vi "Gyro Color Assisted PID C1C2.vi"(4 "Colour 1 threshold":sgl=14.0, 6 "Ini. Degrees":sgl, 7 "Motor":cluster{"Port":T2, "Port":T2}={"Port"=1, "Port"=2} {"Port" items=["Port A", "Port B", "Port C", "Port D"]; "Port" items=["Port A", "Port B", "Port C", "Port D"]}, 9 "De-acc":i32=40, 10 "Acc":i32=80, 11 "EV3 in":T1) -> (3 "EV3 out":T1)   [LabVIEW 2016]
uses:
  <vilib>/NXT/Block Support/NXT_OutputPort.ctl
  <vilib>/NXT/Subs/LVHSConnector.ctl
  <vilib>/NXT/LegoClasses/BrickReference/BrickReference.lvclass
  <vilib>/NXT/Block Support/NXT_InputPort.ctl
  <vilib>/NXT/NXTIO Xnodes/NXTIONodeSubVIs/LEGOResetMotors.vi
  <vilib>/NXT/Dual Mode Library/Sensors/EV3_Gyro_Angle.vi
  <vilib>/NXT/Dual Mode Library/Motors/Rotation.vi
  <vilib>/NXT/Dual Mode Library/Sensors/EV3_Color_Reflect.vi
  <vilib>/NXT/NXTIO Xnodes/NXTIONodeSubVIs/NXTMotorSteeringOn.vi
  <vilib>/NXT/NXTIO Xnodes/NXTIOXNode/NXTIO.xnode
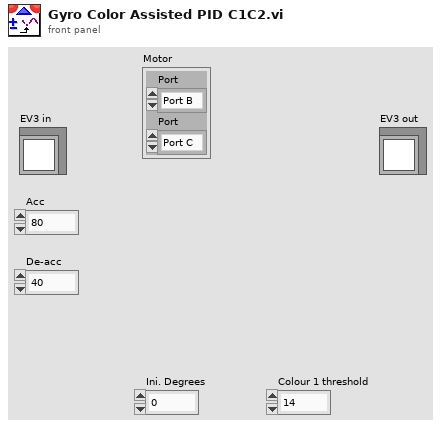
[diagram p1: front panel]
types:
  T1 = typedef "LVHSConnector.ctl" = refnum<class "BrickReference.lvclass">
  T2 = typedef "NXT_OutputPort.ctl" = u8
  T3 = typedef "NXT_InputPort.ctl" = u32
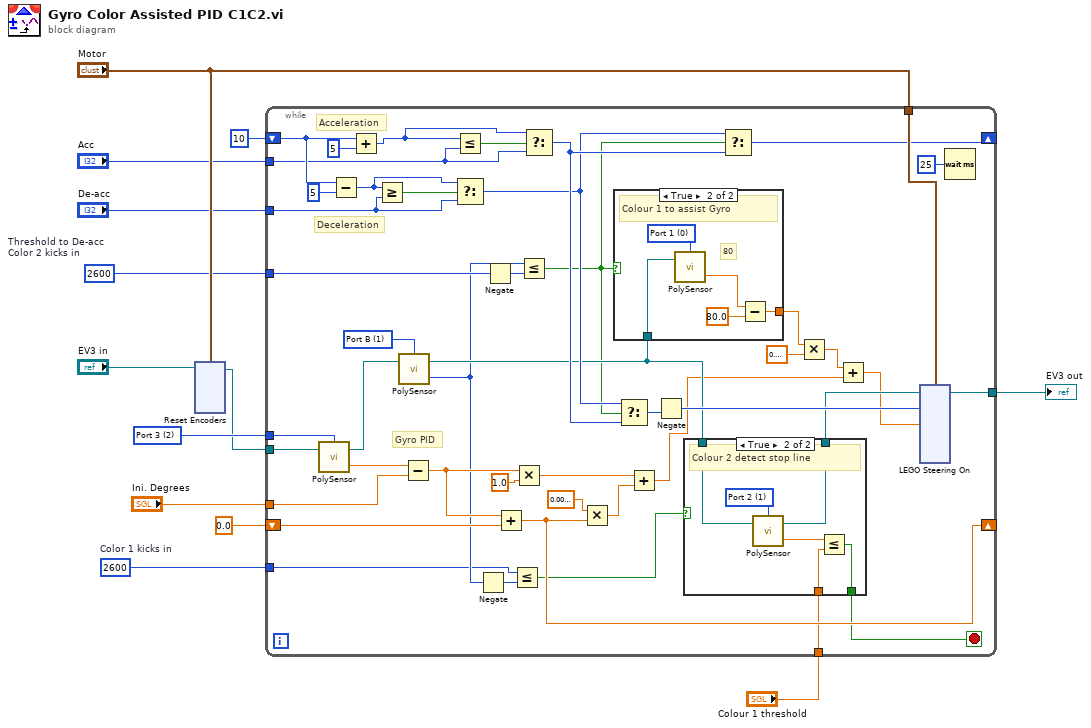
[diagram p0: block diagram]
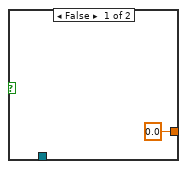
[diagram p2: hidden frame]
diagram:
  w1 = 2600  # Color 1 kicks in
  w3 = 2600  # Threshold to De-acc Color 2 kicks in
  w11 = T3 2 items=["Port 1", "Port 2", "Port 3", "Port 4"] ("Port (Gyro)")
  n1 = xnode "Reset Encoders"("Motors"="Motor", "NXT/EV3"="EV3 in") -> ("NXT/EV3"=w8:T1)
  n2 = while {
    tunnel: w8 -> [w50]
    tunnel: w11 -> [w44]
    shift-right: [w56] -> _
    shift-left: sgl 0.0 -> [w57]
    tunnel: "Ini. Degrees" -> [w52]
    tunnel: [w43] -> w2
    tunnel: "Motor" -> [w49]
    shift-right: [w29] -> _
    shift-left: 10 -> [w34]
    tunnel: "Colour 1 threshold" -> [w28]
    tunnel: "De-acc" -> [w27]
    tunnel: "Acc" -> [w26]
    tunnel: w3 -> [w19]
    tunnel: w1 -> [w14]
    stop <- w36 stop-if-true
    w47 = T2 1 items=["Port A", "Port B", "Port C", "Port D"] ("Port (Port A)")
    # "Acceleration"
    # "Gyro PID"
    # "Deceleration"
    n3 = call-poly <vilib>:"PolySensor.vi"("NXT/EV3"=w50, "Port (Port 1)"=w44) -> ("Degrees"=w59:sgl, "NXT/EV3"=w48:T1)  [unwired: 1 in]
    n4 = Subtract(x=w34, y=5) -> (x-y=w37:i32)
    n5 = Add(x=w34, y=5) -> (x+y=w32:i32)
    n6 = Greater Or Equal?(x=w37, y=w27) -> (x >= y?=w38:bool)
    n7 = call-poly <vilib>:"PolySensor.vi"("NXT/EV3"=w48, "Port (Port A)"=w47) -> ("Angle of Rotation"=w16:i32, "NXT/EV3"=w25:T1)  [unwired: 1 in]
    n8 = Subtract(x=w59, y=w52) -> (x-y=w51:sgl)
    n9 = Less Or Equal?(x=w32, y=w26) -> (x <= y?=w41:bool)
    n10 = Select(t=w37, s=w38, f=w27) -> (s? t:f=w30:i32)
    n11 = Negate(x=w16) -> (-x=w17:i32)
    n12 = Negate(x=w19) -> (-x=w45:i32)
    n13 = Add(x=w51, y=w57) -> (x+y=w56:sgl)
    n14 = Less Or Equal?(x=w14, y=w17) -> (x <= y?=w15:bool)
    n15 = Multiply(x=w51, y=sgl 1.0 ("K_p")) -> (x*y=w54:sgl)
    n16 = Less Or Equal?(x=w16, y=w45) -> (x <= y?=w18:bool)
    n17 = Select(t=w32, s=w41, f=w26) -> (s? t:f=w31:i32)
    n18 = Multiply(x=sgl 0.01 ("K_i"), y=w56) -> (x*y=w53:sgl)
    n19 = case shown="True" w18 {
      tunnel: w25 -> [_ w64]
      tunnel: [sgl 0.0 w63] -> w24
      frame False {
      }
      frame True {
        w65 = T3 0 items=["Port 1", "Port 2", "Port 3", "Port 4"] ("Port (Port 1)")
        # "80"
        # "Colour 1 to assist Gyro"
        n20 = call-poly <vilib>:"PolySensor.vi"("NXT/EV3"=w64, "Port (Port 1)"=w65) -> ("Scaled Value"=w61:sgl)  [unwired: 1 in, 1 out]
        n21 = Subtract(x=w61, y=sgl 80.0) -> (x-y=w63:sgl)
      }
    }
    n22 = Select(t=w30, s=w18, f=w31) -> (s? t:f=w40:i32)
    n23 = Add(x=w54, y=w53) -> (x+y=w21:sgl)
    n24 = Negate(x=w40) -> (-x=w46:i32)
    n25 = case shown="True" w15 {
      tunnel: [_ w70] -> w36
      tunnel: w25 -> [w66 w69]
      tunnel: [w66 w68] -> w35
      tunnel: w28 -> [_ w67]
      frame False {
      }
      frame True {
        w72 = T3 1 items=["Port 1", "Port 2", "Port 3", "Port 4"] ("Port (Port 1)")
        # "Colour 2 detect stop line"
        n26 = call-poly <vilib>:"PolySensor.vi"("NXT/EV3"=w69, "Port (Port 1)"=w72) -> ("Scaled Value"=w71:sgl, "NXT/EV3"=w68:T1)  [unwired: 1 in]
        n27 = Less Or Equal?(x=w71, y=w67) -> (x <= y?=w70:bool)
      }
    }
    n28 = Select(t=w30, s=w18, f=w31) -> (s? t:f=w29:i32)
    n29 = Multiply(x=w24, y=sgl 0.1) -> (x*y=w22:sgl)
    n30 = Add(x=w22, y=w21) -> (x+y=w20:sgl)
    n31 = xnode "LEGO Steering On"("Steering 1"=w20, "Power 1"=w46, "Motors"=w49, "NXT/EV3"=w35) -> ("NXT/EV3"=w43:T1)
    n32 = Wait (ms)(milliseconds to wait=u32 25) -> ()  [unwired: 1 out]
  }
  "EV3 out" <- w2
